vi "Scalar Queue Benchmark.vi"() -> ()   [LabVIEW 2022 SP3]
uses:
  Enclave/Element.ctl
  Enclave/Enclave.lvlib
panel:
  out "El / S":i32(graph)
  out "Element":T1
  in  "stop":bool
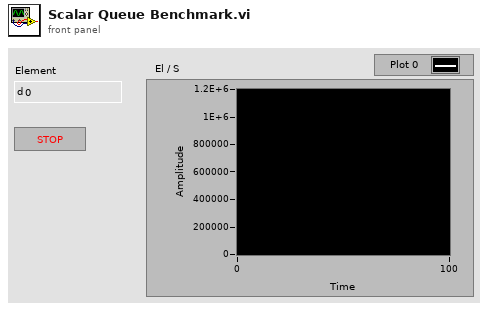
[diagram p1: front panel]
types:
  T1 = typedef "Enclave.lvlib/Element.ctl" = dbl
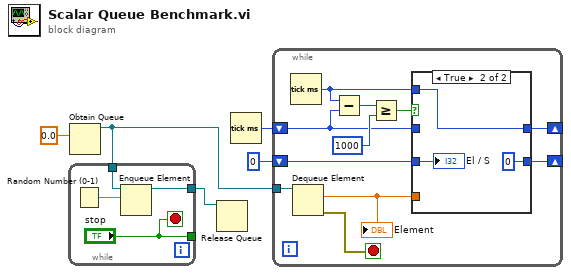
[diagram p0: block diagram]
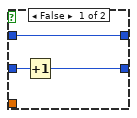
[diagram p2: hidden frame]
diagram:
  n1 = Obtain Queue(element data type=T1 0.0 ("Element")) -> (queue out=w2:refnum<queue>)  [unwired: 4 in, 2 out]
  n2 = while {
    tunnel: ["stop"] -> _
    tunnel: w2 -> [w8]
    tunnel: [w6] -> w1
    stop <- "stop" stop-if-true
    n3 = Random Number (0-1)() -> (number: 0 to 1=w7:dbl)
    n4 = Enqueue Element(queue=w8, element=w7) -> (queue out=w6:refnum<queue>)  [unwired: 2 in, 2 out]
  }
  n5 = Release Queue(queue=w1) -> ()  [unwired: 2 in, 3 out]
  n6 = Tick Count (ms)() -> (millisecond timer value=w5:u32)
  n7 = while {
    tunnel: w2 -> [w12]
    shift-right: [w15] -> _
    shift-left: w5 -> [w18]
    shift-right: [w13] -> _
    shift-left: 0 -> [w14]
    stop <- w10 stop-if-true
    n8 = Tick Count (ms)() -> (millisecond timer value=w16:u32)
    n9 = Dequeue Element(queue=w12) -> (element=w11:T1, error out=w10:errorcluster)  [unwired: 2 in, 2 out]
    "Element" <- w11
    n10 = Subtract(x=w16, y=w18) -> (x-y=w20:u32)
    n11 = Greater Or Equal?(x=w20, y=u32 1000) -> (x >= y?=w17:bool)
    n12 = case shown="True" w17 {
      tunnel: w18 -> [w23 _]
      tunnel: w16 -> [_ w26]
      tunnel: [w23 w26] -> w15
      tunnel: w14 -> [w22 w25]
      tunnel: [w21 0] -> w13
      tunnel: w11 -> [_ _]
      frame False {
        n13 = Increment(x=w22) -> (x+1=w21:i32)
      }
      frame True {
        "El / S" <- w25
      }
    }
  }
